vi "TH_TelldusLiveParser.vi"(0 "Telldus Sensor String":string, 11 "error in (no error)":errorcluster) -> (3 "Name":string, 4 "Temperature":dbl format="%.1g", 6 "Humidity":dbl format="%.1g", 8 "Date":string, 10 "Time":string, 15 "error out":errorcluster)   [LabVIEW 2014]
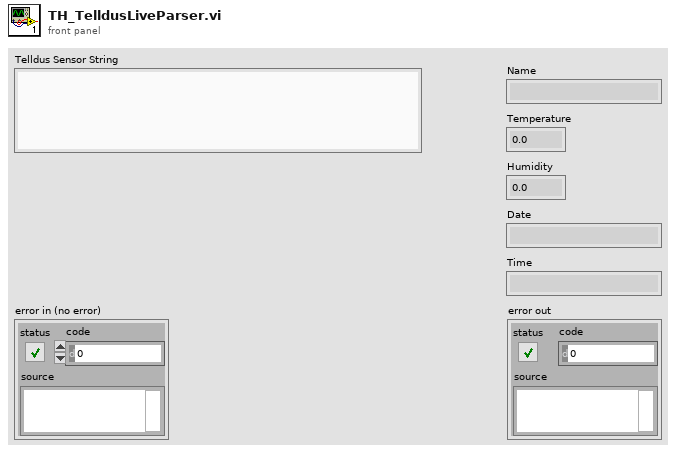
[diagram p1: front panel]
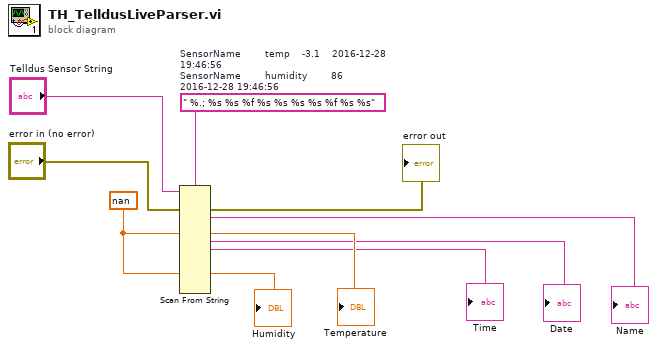
[diagram p0: block diagram]
diagram:
  w4 = nan
  w8 = " %.; %s %s %f %s %s %s %s %f %s %s"  # SensorName        temp    -3.1    2016-12-28 19:46:56 SensorName        humidity        86      2016-12-28 19:46:56
  n1 = Scan From String(format string=w8, input string="Telldus Sensor String", error in="error in (no error)", default 3=w4, default 8=w4) -> (error out=→"error out":errorcluster, output 1=→"Name":string, output 3=→"Temperature":dbl, output 4=→"Date":string, output 5=→"Time":string, output 8=→"Humidity":dbl)  [unwired: 14 in, 2 out]
